vi "Get PID Parameters.vi"(2 "gain scheduling":T1={"gain schedule"=[100.0], "PID parameters"=[{"Kc"=0.0, "Ti (min)"=0.0, "Td (min)"=0.0}], "scheduling input"=0} {"scheduling input" items=["Setpoint", "Process variable", "Controller output", "Gain scheduling input"]; "PID parameters"."Td (min)" format="%.4f"; "PID parameters"."Ti (min)" format="%.4f"; "PID parameters"."Kc" format="%.4f"; "gain schedule" format="%.2f"}, 3 "scheduling variable":dbl format="%.2f") -> (0 "scheduling index":i32, 1 "PID parameters":cluster{"Kp":dbl, "Ti":dbl, "Td":dbl} {"Td" format="%.2f"; "Ti" format="%.2f"; "Kp" format="%.2f"})   [LabVIEW 2017, in "NI_PID__autopid compat.lvlib"]
doc: "This VI selects the PID gains to be used from the gain schedule."
uses:
  <vilib>/addons/control/pid/NI_PID__autopid compat.lvlib
panel:
  # "Get PID Parameters"
  # "Proportional gain or band (Kc)"
  # "Integral (reset) time (Ti, min)"
  # "Derivative (rate) time (Td, min)"
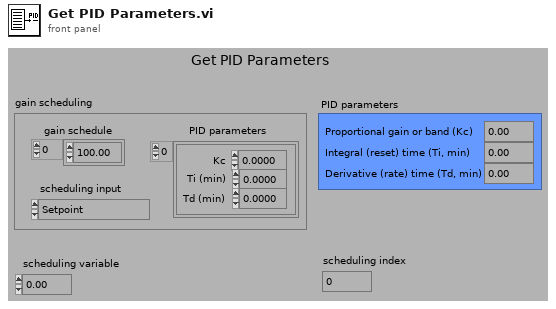
[diagram p1: front panel]
types:
  T1 = cluster{"gain schedule":dbl[], "PID parameters":cluster{"Kc":dbl, "Ti (min)":dbl, "Td (min)":dbl}[], "scheduling input":u16}
  T2 = cluster{"Kc":dbl, "Ti (min)":dbl, "Td (min)":dbl}[]
  T3 = cluster{"Kc":dbl, "Ti (min)":dbl, "Td (min)":dbl}
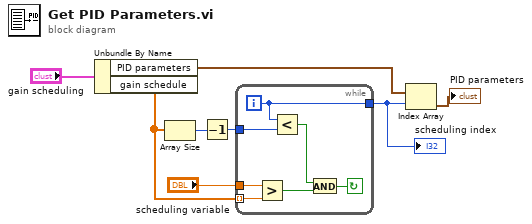
[diagram p0: block diagram]
diagram:
  n1 = Unbundle By Name("gain scheduling") -> ("PID parameters"=w8:T2, "gain schedule"=w3:dbl[])
  n2 = Array Size(array=w3) -> (size(s)=w2:i32)
  n3 = Decrement(x=w2) -> (x-1=w1:i32)
  n4 = while {
    tunnel: w1 -> [w13]
    tunnel: "scheduling variable" -> [w14]
    tunnel: [w12] -> w7
    tunnel: w3 -> [w15] mode=indexing
    i -> [w12]
    stop <- w9 continue-if-true
    n5 = Greater?(x=w14, y=w15) -> (0:w11:bool)
    n6 = Less?(x=w12, y=w13) -> (x < y?=w10:bool)
    n7 = And(x=w10, y=w11) -> (x .and. y?=w9:bool)
  }
  "scheduling index" <- w7
  n8 = Index Array(array=w8, index=w7) -> (element=→"PID parameters":T3)
